vi "Untitled 2.vi"() -> ()   [LabVIEW 2011]
panel:
  in  "Ring 2":u16(ring) items=["Add.vi", "Subtract.vi", "Multiple.vi", "Divide.vi", "Max.vi"]
  out "output":dbl
  in  "Y":dbl
  in  "X":dbl
  in  "stop":bool
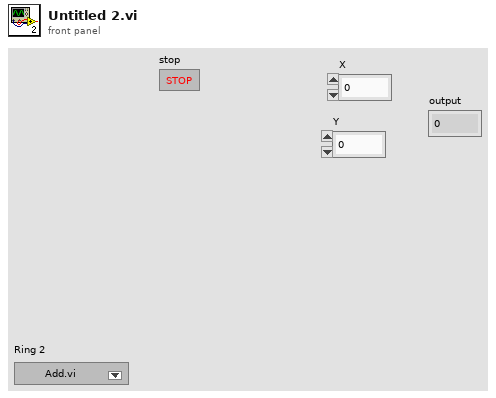
[diagram p1: front panel]
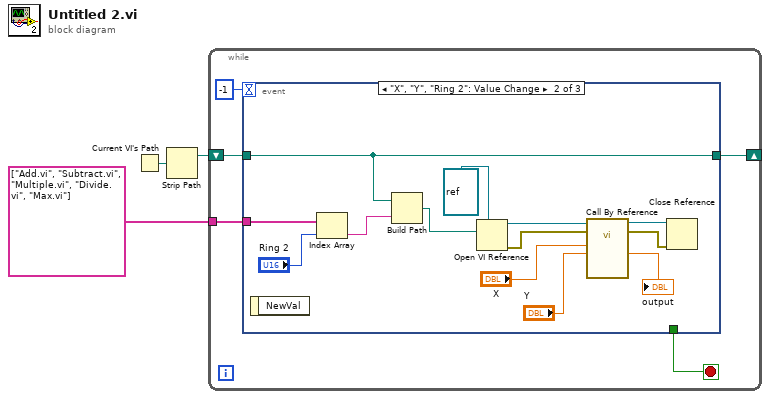
[diagram p0: block diagram]
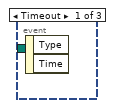
[diagram p2: hidden frame]
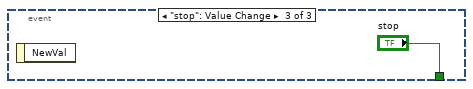
[diagram p3: hidden frame]
diagram:
  n1 = Current VI's Path() -> (path=w2:path)
  n2 = Strip Path(path=w2) -> (stripped path=w1:path)  [unwired: 1 out]
  n3 = while {
    tunnel: string[] ["Add.vi", "Subtract.vi", "Multiple.vi", "Divide.vi", "Max.vi"] -> [w8]
    shift-right: [w6] -> _
    shift-left: w1 -> [w7]
    stop <- w5 stop-if-true
    n4 = event shown="[1] \"X\", \"Y\", \"Ring 2\": Value Change" {
      selector: _ -> [_ _ _]
      dyn-events: _ -> [_ _ _]
      timeout: -1 -> [_ _ _]
      tunnel: w8 -> [_ w21 _]
      tunnel: w7 -> [_ w20 _]
      tunnel: [_ w20 _] -> w6
      tunnel: [_ _ "stop"] -> w5
      event Timeout {
        n5 = event-data() -> ()  [unwired: 1 in, 2 out]
      }
      event "X", "Y", "Ring 2": Value Change {
        n6 = event-data() -> ()  [unwired: 1 in, 1 out]
        n7 = Index Array(array=w21, index="Ring 2") -> (element=w19:string)
        n8 = Build Path(base path=w20, name or relative path=w19) -> (appended path=w18:path)
        n9 = Open VI Reference(type specifier VI Refnum (for type only)=refnum<vi> refnum, vi path=w18) -> (vi reference=w16:refnum<vi>, error out=w15:errorcluster)  [unwired: 4 in]
        n10 = call-by-ref "?"(reference=w16, error in=w15, "input2"="Y", "input1"="X") -> (reference out=w14:refnum<vi>, error out=w13:errorcluster, "output"=→"output":dbl)  [unwired: 8 in, 1 out]
        n11 = Close Reference(reference=w14, error in (no error)=w13) -> ()  [unwired: 1 out]
      }
      event "stop": Value Change {
        n12 = event-data() -> ()  [unwired: 1 in, 1 out]
      }
    }
  }
